vi "MGCC_FntStaMach_Interrupt_1min.vi"() -> (2 "Boolean 2":bool)   [LabVIEW 2016]
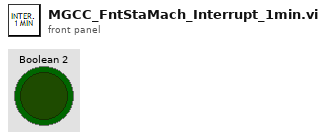
[diagram p1: front panel]
types:
  T1 = cluster{"V_node":cdb[][], "P_node":cdb[][], "I_node":cdb[][], "NumN":dbl, "NumL":dbl, "Ybus":cdb[][], "sspn":dbl[][], "ssqn":dbl[][], "ssvn":dbl[][], "SlackBus":dbl, "Topology":dbl[][]}
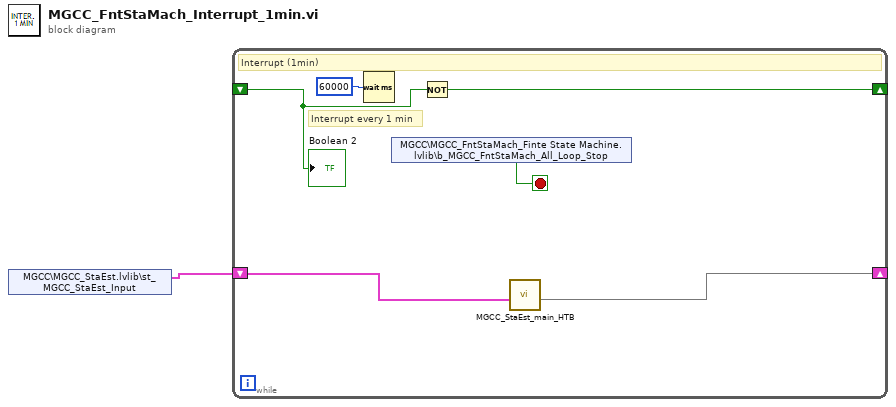
[diagram p0: block diagram]
diagram:
  n1 = shared-variable "MGCC\\MGCC_StaEst.lvlib\\st_MGCC_StaEst_Input"() -> (w1:T1)  [unwired: 1 in, 1 out]
  n2 = while {
    shift-right: [w6] -> _
    shift-left: _ -> [w5]
    shift-right: [w3] -> _
    shift-left: w1 -> [w2]
    stop <- w4 stop-if-true
    # "Interrupt every 1 min"
    # "Interrupt (1min)"
    n3 = Wait (ms)(milliseconds to wait=u32 60000) -> ()  [unwired: 1 out]
    n4 = shared-variable "MGCC\\MGCC_FntStaMach_Finte State Machine.lvlib\\b_MGCC_FntStaMach_All_Loop_Stop"() -> (w4:bool)  [unwired: 1 in, 1 out]
    n5 = Not(x=w5) -> (.not. x?=w6:bool)
    n6 = call "MGCC_StaEst_main_HTB.vi"(9:w2) -> (1:w3)  [unwired: 10 in]
    "Boolean 2" <- w5
  }
